vi "createUserEditableAmount.vi"(8 "error in (no error)":errorcluster, 10 "Create":dbl, 11 "UserEditableAmount":refnum<class "UserEditableAmount.lvclass">) -> (0 "error out":errorcluster, 3 "UserEditableAmount out":refnum<class "UserEditableAmount.lvclass">)   [LabVIEW 2018, in "UserEditableAmount.lvclass"]
uses:
  UserEditableAmount.lvclass
  UserEditableAmount.lvclass/UserEditableAmount.ctl
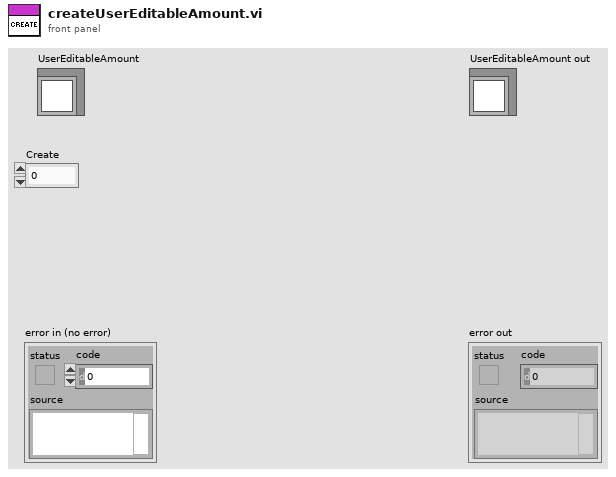
[diagram p1: front panel]
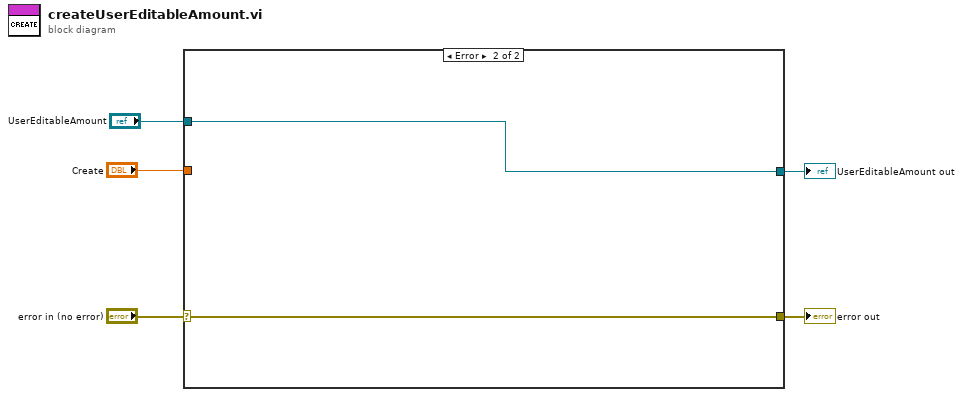
[diagram p0: block diagram]
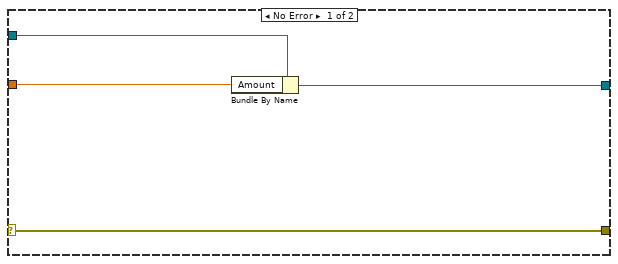
[diagram p2: hidden frame]
diagram:
  n1 = case shown="Error" "error in (no error)" {
    selector: "error in (no error)" -> [w9 w11]
    tunnel: [w9 w11] -> w4
    tunnel: [w7 w10] -> w3
    tunnel: "Create" -> [w8 _]
    tunnel: "UserEditableAmount" -> [w6 w10]
    frame No Error {
      n2 = Bundle By Name(cluster=w6, "Amount"=w8) -> (w7:refnum<class "UserEditableAmount.lvclass">)
    }
    frame Error {
    }
  }
  "error out" <- w4
  "UserEditableAmount out" <- w3
